vi "Run Till Stable2.vi"(11 "output cluster":T1) -> (1 "Boolean":bool, 2 "Delta":dbl, 3 "Array":dbl[](array[numeric]))   [LabVIEW 2016]
uses:
  Controls/Cal Refs.ctl
  <vilib>/Analysis/baseanly.llb/Mean (DBL).vi
  <vilib>/Analysis/NI_AALBase.lvlib
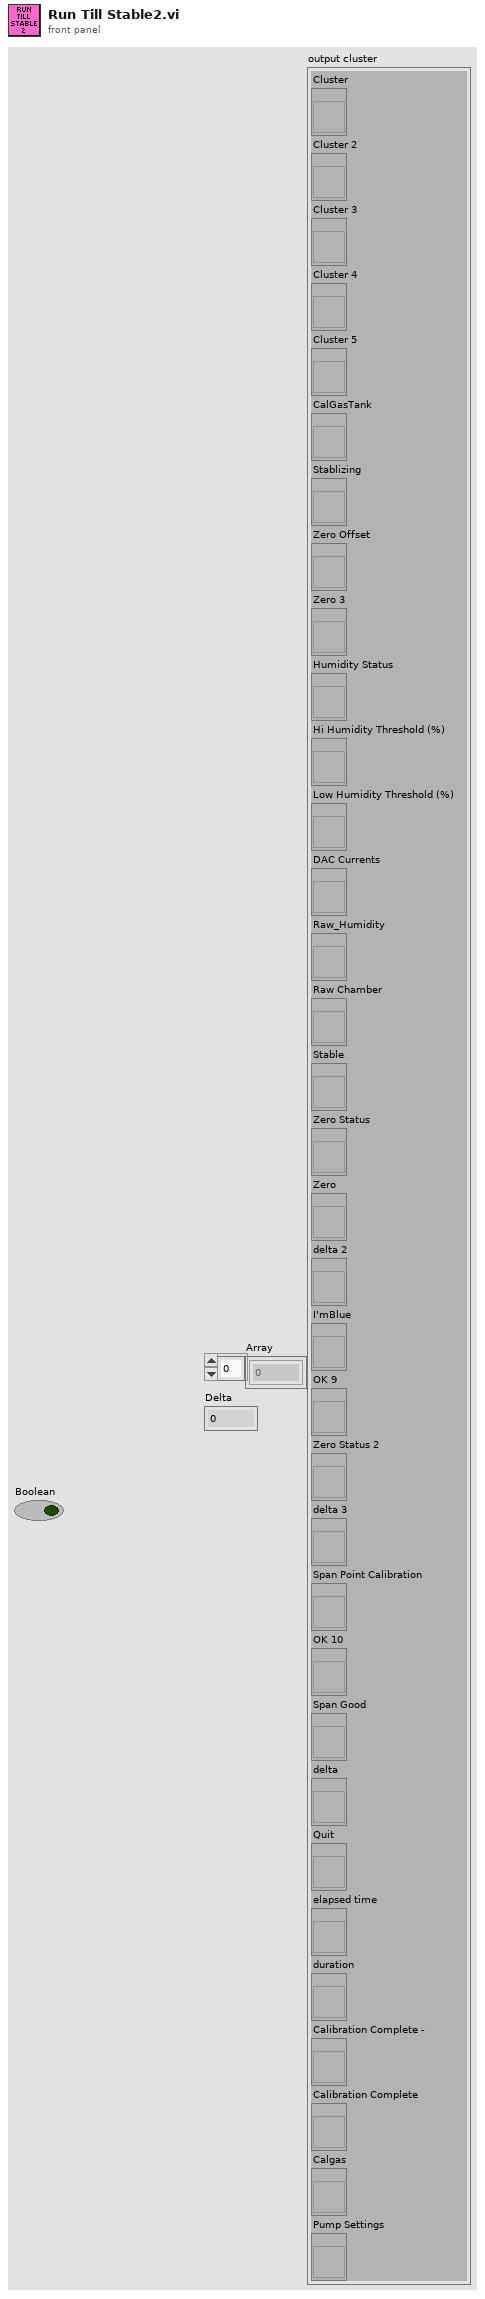
[diagram p1: front panel]
types:
  T1 = typedef "Cal Refs.ctl" = cluster{"Cluster":refnum<vi>, "Cluster 2":refnum<vi>, "Cluster 3":refnum<vi>, "Cluster 4":refnum<vi>, "Cluster 5":refnum<vi>, "CalGasTank":refnum<vi>, "Stablizing":refnum<vi>, "Zero Offset":refnum<vi>, "Zero 3":refnum<vi>, "Humidity Status":refnum<vi>, "Hi Humidity Threshold (%)":refnum<vi>, "Low Humidity Threshold (%)":refnum<vi>, "DAC Currents":refnum<vi>, "Raw_Humidity":refnum<vi>, "Raw Chamber":refnum<vi>, "Stable":refnum<vi>, "Zero Status":refnum<vi>, "Zero":refnum<vi>, "delta 2":refnum<vi>, "I'mBlue":refnum<vi>, "OK 9":refnum<vi>, "Zero Status 2":refnum<vi>, "delta 3":refnum<vi>, "Span Point Calibration":refnum<vi>, "OK 10":refnum<vi>, "Span Good":refnum<vi>, "delta":refnum<vi>, "Quit":refnum<vi>, "elapsed time":refnum<vi>, "duration":refnum<vi>, "Calibration Complete -":refnum<vi>, "Calibration Complete":refnum<vi>, "Calgas":refnum<vi>, "Pump Settings":refnum<vi>}
  T2 = cluster{"Tcal_Chamber":dbl, "Tcal_PCB":dbl, "Tcal_Film":dbl, "Tcal_Humidity":dbl, "Tcal_Det":dbl[], "Cal Gas":dbl, "Reference":dbl}
  T3 = cluster{"CalFile Selected":path, "TYPE":string, "DATE":string, "C0FC2V":dbl[], "C6FC2V":dbl[], "V_0d(target)":dbl[], "V_6d(target)":dbl[], "V_span(target)":dbl[], "CHANNEL":string[], "Status":bool[], "BlueLED 2":bool[], "C2V":u8[], "A":dbl[], "B":dbl[], "C":dbl[], "D":dbl[], "V2C":u8[], "A'":dbl[], "B'":dbl[], "C'":dbl[], "D'":dbl[]}
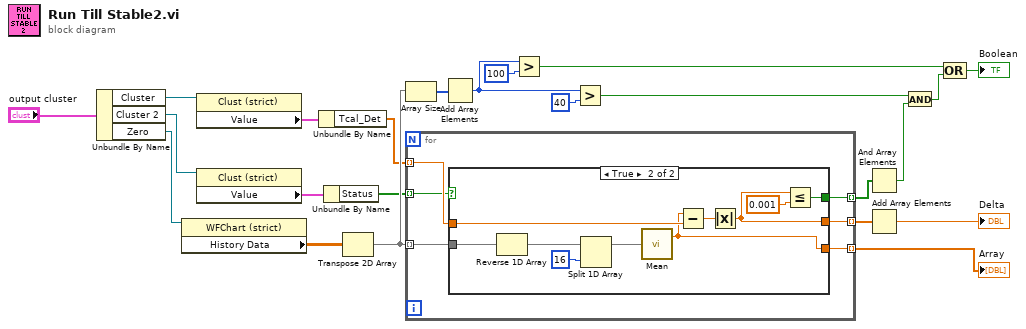
[diagram p0: block diagram]
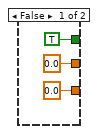
[diagram p2: hidden frame]
diagram:
  n1 = Unbundle By Name("output cluster") -> ("Cluster"=w5:refnum<vi>, "Cluster 2"=w9:refnum<vi>, "Zero"=w2:refnum<vi>)
  n2 = property on="Property Node" class="WFChart (strict)"(reference=w2) -> ("History Data"=w14:dbl[][])  [unwired: 1 in, 2 out]
  n3 = property class="Clust (strict)"(reference=w5) -> ("Value"=w7:T2)  [unwired: 1 in, 2 out]
  n4 = property class="Clust (strict)"(reference=w9) -> ("Value"=w8:T3)  [unwired: 1 in, 2 out]
  n5 = Unbundle By Name(w7) -> ("Tcal_Det"=w4:dbl[])
  n6 = Unbundle By Name(w8) -> ("Status"=w3:bool[])
  n7 = Transpose 2D Array(2D array=w14) -> (transposed array=w15:dbl[][])
  n8 = Array Size(array=w15) -> (size(s)=w10:i32[])
  n9 = for {
    tunnel: w15 -> [w29] mode=indexing
    tunnel: w4 -> [w28] mode=indexing
    tunnel: [w27] -> w16 mode=indexing
    tunnel: [w26] -> w23 mode=indexing
    tunnel: [w25] -> w22 mode=indexing
    tunnel: w3 -> [w24] mode=indexing
    n10 = case shown="True" w24 {
      tunnel: w29 -> [_ w37]
      tunnel: w28 -> [_ w36]
      tunnel: [TRUE w35] -> w27
      tunnel: [0.0 ("mean") w34] -> w26
      tunnel: [0.0 w33] -> w25
      frame False {
      }
      frame True {
        n11 = Reverse 1D Array(array=w37) -> (reversed array=w38:dbl[])
        n12 = Split 1D Array(array=w38, index=16) -> (first subarray=w39:dbl[])  [unwired: 1 out]
        n13 = call-poly <vilib>:"Mean.vi"("X"=w39) -> ("mean"=w34:dbl)  [unwired: 1 out]
        n14 = Subtract(x=w34, y=w36) -> (x-y=w41:dbl)
        n15 = Absolute Value(x=w41) -> (abs(x)=w33:dbl)
        n16 = Less Or Equal?(x=w33, y=0.001) -> (x <= y?=w35:bool)
      }
    }
  }
  "Array" <- w23
  n17 = Add Array Elements(numeric array=w10) -> (sum=w20:i32)
  n18 = Greater?(x=w20, y=100 ("index")) -> (0:w21:bool)
  n19 = Greater?(x=w20, y=40 ("index")) -> (0:w12:bool)
  n20 = And Array Elements(Boolean array=w16) -> (logical AND=w17:bool)
  n21 = Add Array Elements(numeric array=w22) -> (sum=→"Delta":dbl)
  n22 = And(x=w12, y=w17) -> (x .and. y?=w18:bool)
  n23 = Compound Arithmetic op=OR(w21, w18) -> (→"Boolean":bool)
